vi "verify parameters in range.vi"(8 "error in (no error)":errorcluster, 11 "Simulated_CCD_Camera in":refnum<class "Simulated_CCD_Camera.lvclass">) -> (0 "error out":errorcluster, 3 "Simulated_CCD_Camera out":refnum<class "Simulated_CCD_Camera.lvclass">)   [LabVIEW 2018, in "Simulated_CCD_Camera.lvclass"]
uses:
  Simulated_CCD_Camera.lvclass
  Simulated_CCD_Camera.lvclass/Simulated_CCD_Camera.ctl
  <vilib>/ErrorRing/Error Ring.xnode
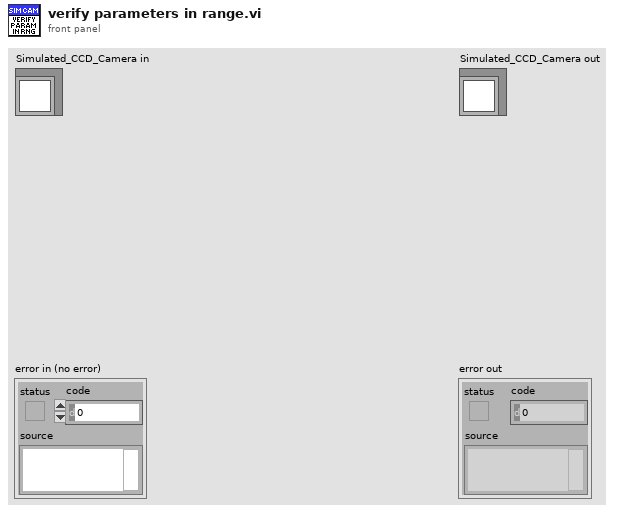
[diagram p1: front panel]
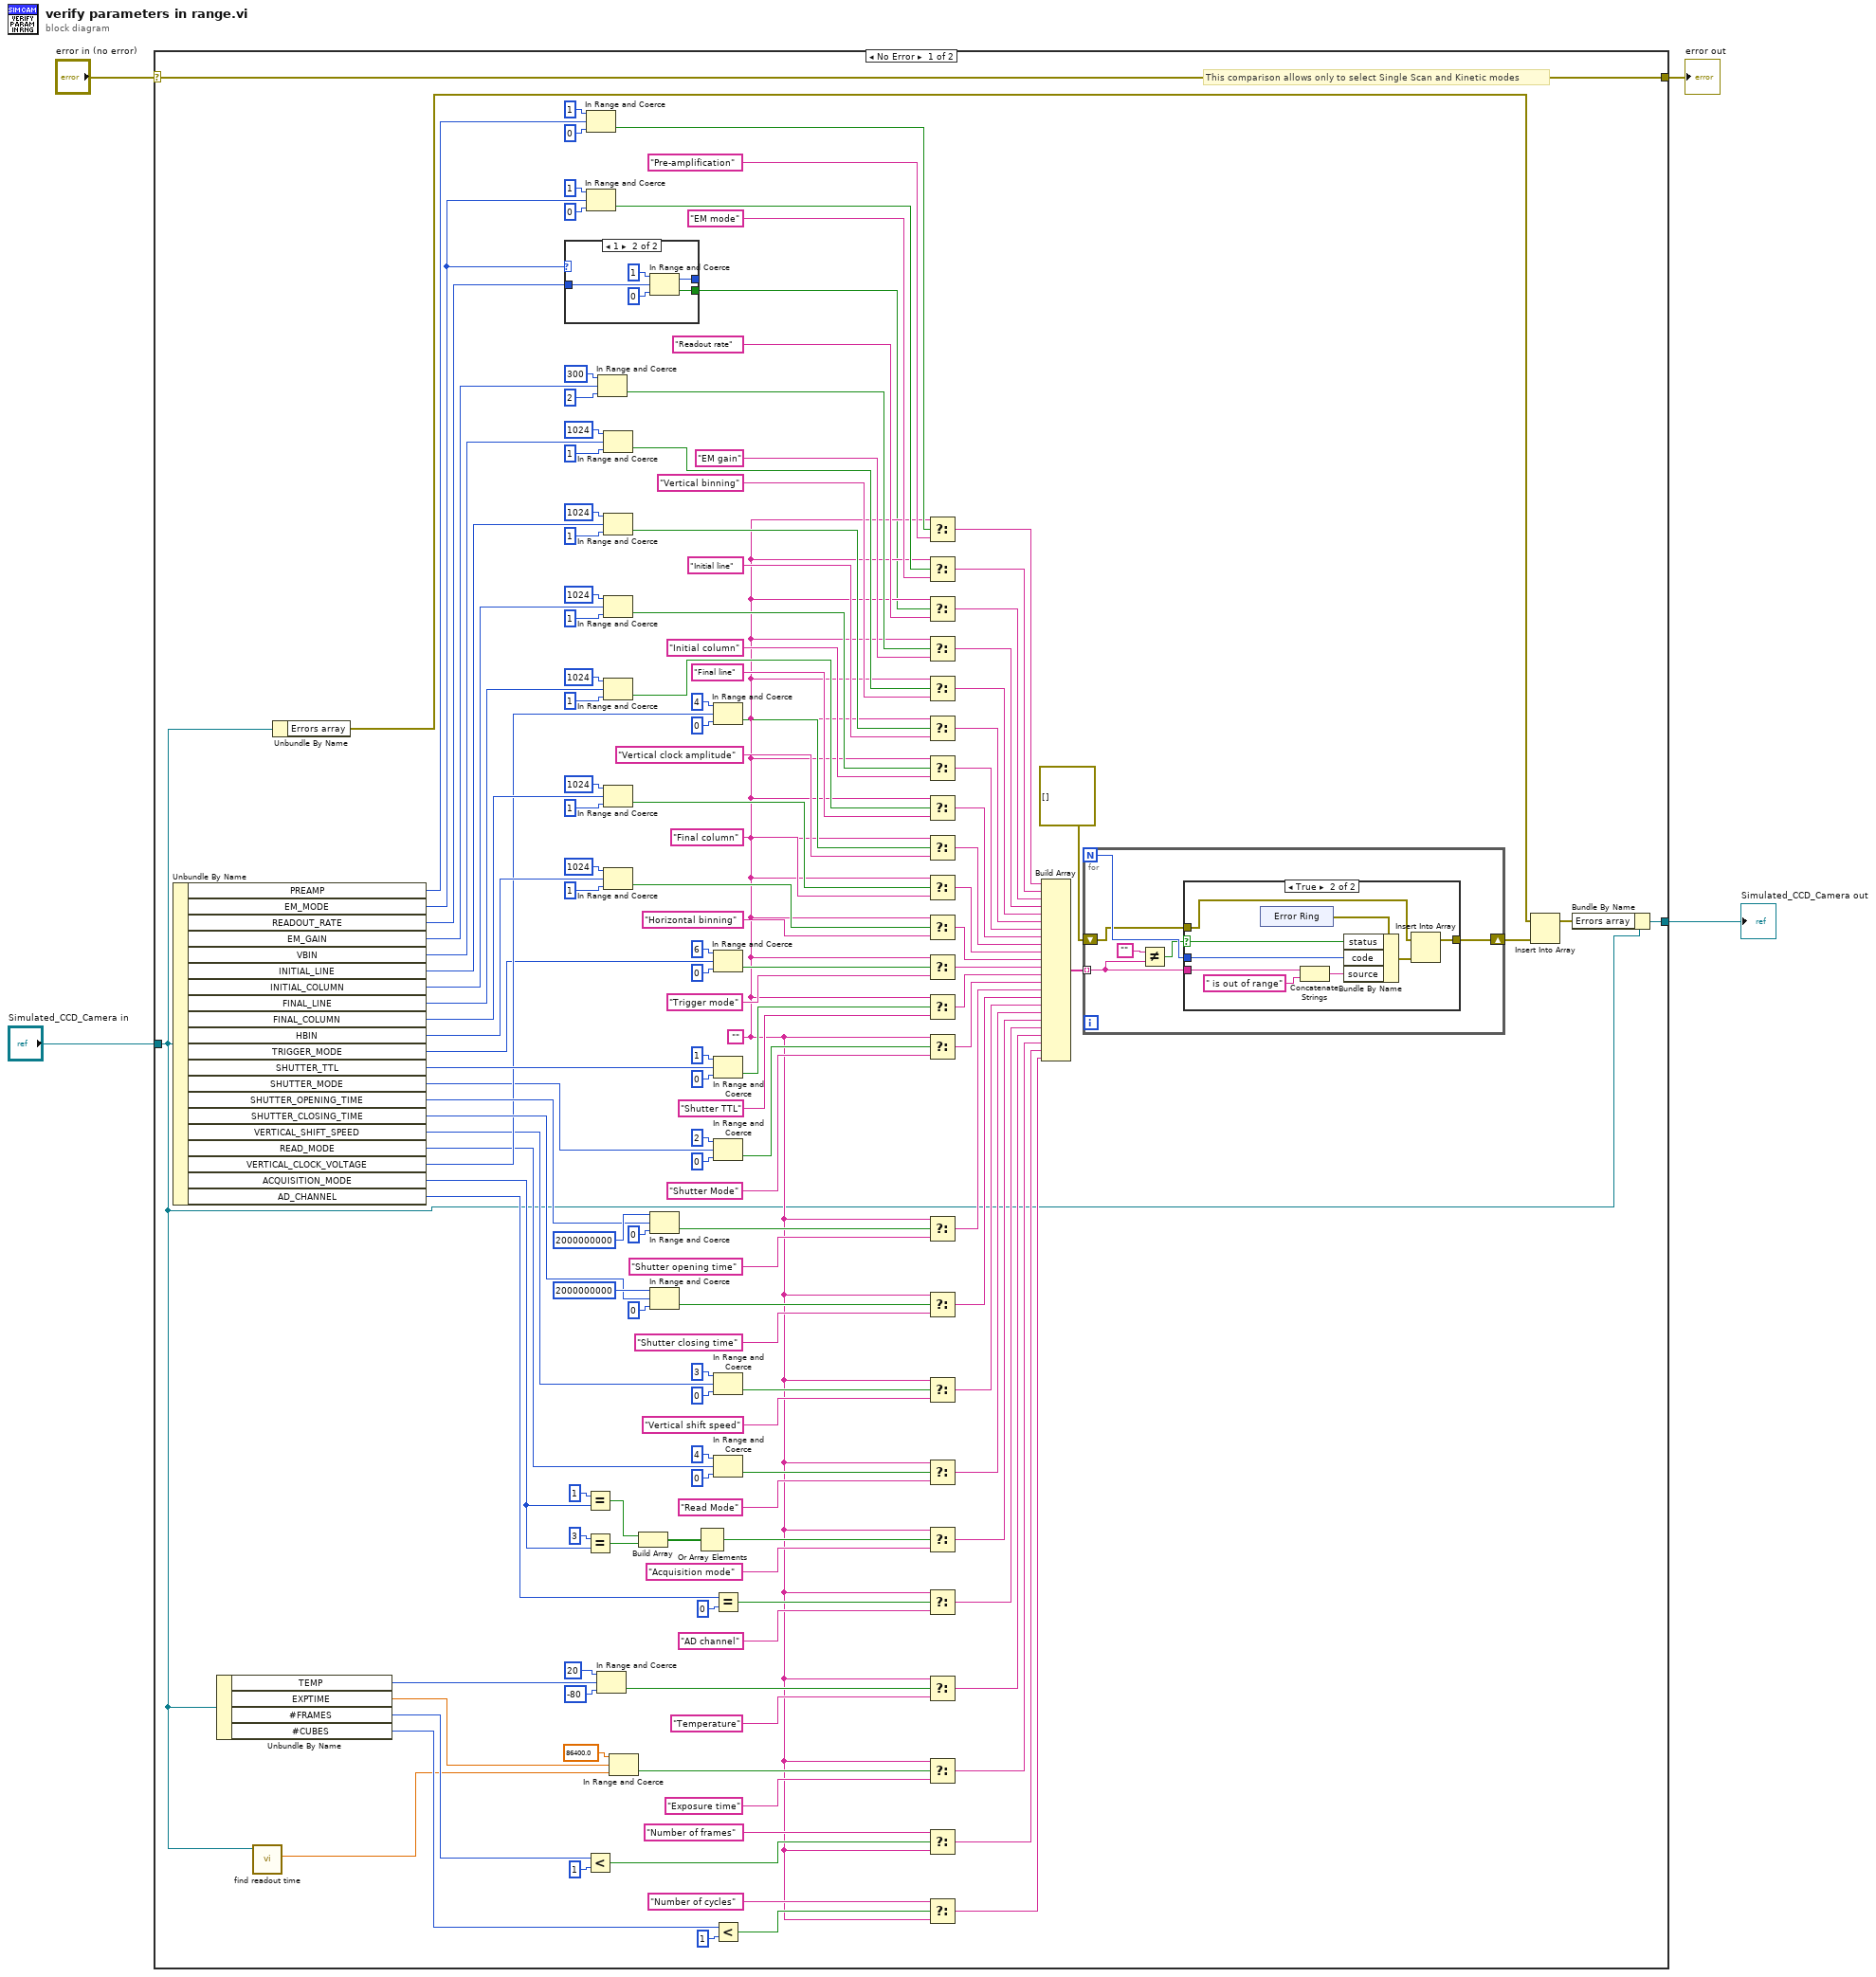
[diagram p0: block diagram]
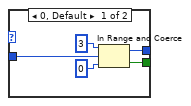
[diagram p3: hidden frame]
diagram:
  n1 = case shown="No Error" "error in (no error)" {
    selector: "error in (no error)" -> [w102 w184]
    tunnel: [w102 w184] -> w3
    tunnel: [w14 w183] -> w1
    tunnel: "Simulated_CCD_Camera in" -> [w6 w183]
    frame No Error {
      w15 = ""
      # "This comparison allows only to select Single Scan and Kinetic modes"
      n2 = Unbundle By Name(w6) -> ("PREAMP"=w153:u16, "EM_MODE"=w150:u16, "READOUT_RATE"=w149:u16, "EM_GAIN"=w146:u16, "VBIN"=w143:u16, "INITIAL_LINE"=w140:u16, "INITIAL_COLUMN"=w137:u16, "FINAL_LINE"=w134:u16, "FINAL_COLUMN"=w131:u16, "HBIN"=w128:u16, "TRIGGER_MODE"=w103:u16, "SHUTTER_TTL"=w125:u16, "SHUTTER_MODE"=w111:u16, "SHUTTER_OPENING_TIME"=w122:u16, "SHUTTER_CLOSING_TIME"=w119:u16, "VERTICAL_SHIFT_SPEED"=w108:u16, "READ_MODE"=w105:u16, "VERTICAL_CLOCK_VOLTAGE"=w116:u16, "ACQUISITION_MODE"=w49:u16, "AD_CHANNEL"=w41:u16)
      n3 = Unbundle By Name(w6) -> ("TEMP"=w34:i32, "EXPTIME"=w29:dbl, "#FRAMES"=w25:u32, "#CUBES"=w20:u32)
      n4 = call "find readout time.vi"("Simulated_CCD_Camera in"=w6) -> ("readout time"=w5:dbl)  [unwired: 8 in, 2 out]
      n5 = Unbundle By Name(w6) -> ("Errors array"=w10:errorcluster[])
      n6 = case shown="1" w150 {
        tunnel: w149 -> [w175 w180]
        tunnel: [w174 w179] -> _
        tunnel: [w173 w178] -> w7
        frame 0, Default {
          n7 = In Range and Coerce(upper limit=3, x=w175, lower limit=0) -> (coerced(x)=w174:i32, In Range?=w173:bool)
        }
        frame 1 {
          n8 = In Range and Coerce(upper limit=1, x=w180, lower limit=0) -> (coerced(x)=w179:i32, In Range?=w178:bool)
        }
      }
      n9 = Equal?(x=1, y=w49) -> (x = y?=w46:bool)
      n10 = Equal?(x=3, y=w49) -> (x = y?=w47:bool)
      n11 = Less?(x=w25, y=1) -> (x < y?=w23:bool)
      n12 = In Range and Coerce(upper limit=1, x=w153, lower limit=0) -> (In Range?=w97:bool)  [unwired: 1 out]
      n13 = In Range and Coerce(upper limit=1, x=w150, lower limit=0) -> (In Range?=w96:bool)  [unwired: 1 out]
      n14 = In Range and Coerce(upper limit=20, x=w34, lower limit=-80) -> (In Range?=w33:bool)  [unwired: 1 out]
      n15 = In Range and Coerce(upper limit=300, x=w146, lower limit=2) -> (In Range?=w93:bool)  [unwired: 1 out]
      n16 = In Range and Coerce(upper limit=1024, x=w143, lower limit=1) -> (In Range?=w90:bool)  [unwired: 1 out]
      n17 = In Range and Coerce(upper limit=1024, x=w140, lower limit=1) -> (In Range?=w85:bool)  [unwired: 1 out]
      n18 = In Range and Coerce(upper limit=1024, x=w137, lower limit=1) -> (In Range?=w84:bool)  [unwired: 1 out]
      n19 = In Range and Coerce(upper limit=1024, x=w134, lower limit=1) -> (In Range?=w81:bool)  [unwired: 1 out]
      n20 = In Range and Coerce(upper limit=1024, x=w131, lower limit=1) -> (In Range?=w77:bool)  [unwired: 1 out]
      n21 = In Range and Coerce(upper limit=1024, x=w128, lower limit=1) -> (In Range?=w74:bool)  [unwired: 1 out]
      n22 = In Range and Coerce(upper limit=86400.0, x=w29, lower limit=w5) -> (In Range?=w28:bool)  [unwired: 1 out]
      n23 = Build Array(w46, w47) -> (w45:bool[])
      n24 = In Range and Coerce(upper limit=2000000000, x=w122, lower limit=0) -> (In Range?=w62:bool)  [unwired: 1 out]
      n25 = In Range and Coerce(upper limit=2000000000, x=w119, lower limit=0) -> (In Range?=w59:bool)  [unwired: 1 out]
      n26 = Or Array Elements(Boolean array=w45) -> (logical OR=w44:bool)
      n27 = In Range and Coerce(upper limit=4, x=w116, lower limit=0) -> (In Range?=w51:bool)  [unwired: 1 out]
      n28 = In Range and Coerce(upper limit=6, x=w103, lower limit=0) -> (In Range?=w72:bool)  [unwired: 1 out]
      n29 = In Range and Coerce(upper limit=1, x=w125, lower limit=0) -> (In Range?=w69:bool)  [unwired: 1 out]
      n30 = In Range and Coerce(upper limit=2, x=w111, lower limit=0) -> (In Range?=w66:bool)  [unwired: 1 out]
      n31 = In Range and Coerce(upper limit=3, x=w108, lower limit=0) -> (In Range?=w57:bool)  [unwired: 1 out]
      n32 = In Range and Coerce(upper limit=4, x=w105, lower limit=0) -> (In Range?=w54:bool)  [unwired: 1 out]
      n33 = Equal?(x=w41, y=0) -> (x = y?=w39:bool)
      n34 = Less?(x=w20, y=1) -> (x < y?=w19:bool)
      n35 = Select(t=w15, s=w97, f="Pre-amplification") -> (s? t:f=w99:string)
      n36 = Select(t=w15, s=w96, f="EM mode") -> (s? t:f=w98:string)
      n37 = Select(t=w15, s=w7, f="Readout rate") -> (s? t:f=w94:string)
      n38 = Select(t=w15, s=w93, f="EM gain") -> (s? t:f=w91:string)
      n39 = Select(t=w15, s=w90, f="Vertical binning") -> (s? t:f=w88:string)
      n40 = Select(t=w15, s=w85, f="Initial line") -> (s? t:f=w86:string)
      n41 = Select(t=w15, s=w84, f="Initial column") -> (s? t:f=w82:string)
      n42 = Select(t=w15, s=w81, f="Final line") -> (s? t:f=w79:string)
      n43 = Select(t=w15, s=w51, f="Vertical clock amplitude") -> (s? t:f=w11:string)
      n44 = Select(t=w15, s=w77, f="Final column") -> (s? t:f=w76:string)
      n45 = Select(t=w15, s=w74, f="Horizontal binning") -> (s? t:f=w73:string)
      n46 = Select(t=w15, s=w72, f="Trigger mode") -> (s? t:f=w70:string)
      n47 = Select(t=w15, s=w69, f="Shutter TTL") -> (s? t:f=w67:string)
      n48 = Select(t=w15, s=w66, f="Shutter Mode") -> (s? t:f=w64:string)
      n49 = Select(t=w15, s=w62, f="Shutter opening time") -> (s? t:f=w61:string)
      n50 = Select(t=w15, s=w59, f="Shutter closing time") -> (s? t:f=w58:string)
      n51 = Select(t=w15, s=w57, f="Vertical shift speed") -> (s? t:f=w55:string)
      n52 = Select(t=w15, s=w54, f="Read Mode") -> (s? t:f=w52:string)
      n53 = Select(t=w15, s=w44, f="Acquisition mode") -> (s? t:f=w42:string)
      n54 = Select(t=w15, s=w39, f="AD channel") -> (s? t:f=w37:string)
      n55 = Select(t=w15, s=w33, f="Temperature") -> (s? t:f=w31:string)
      n56 = Select(t=w15, s=w28, f="Exposure time") -> (s? t:f=w26:string)
      n57 = Select(t="Number of frames" ("f"), s=w23, f=w15) -> (s? t:f=w22:string)
      n58 = Select(t="Number of cycles" ("f"), s=w19, f=w15) -> (s? t:f=w18:string)
      n59 = Build Array(w99, w98, w94, w91, w88, w86, w82, w79, w11, w76, w73, w70, w67, w64, w61, w58, w55, w52, w42, w37, w31, w26, w22, w18) -> (w12:string[])
      n60 = for {
        N -> [w161]
        shift-right: [w160] -> w8
        shift-left: errorcluster[] [] -> [w159]
        tunnel: w12 -> [w156] mode=indexing
        n61 = Not Equal?(x="", y=w156) -> (x != y?=w157:bool)
        n62 = case shown="True" w157 {
          selector: w157 -> [_ w171]
          tunnel: w161 -> [_ w170]
          tunnel: [w162 w169] -> w160
          tunnel: w159 -> [w162 w167]
          tunnel: w156 -> [_ w165]
          frame False {
          }
          frame True {
            n63 = xnode "Error Ring"() -> ("error out"=w168:errorcluster)
            n64 = Concatenate Strings(w165, " is out of range" ("string")) -> (w163:string)
            n65 = Bundle By Name(cluster=w168, "status"=w171, "code"=w170, "source"=w163) -> (w166:errorcluster)
            n66 = Insert Into Array(array=w167, new element=w166) -> (w169:errorcluster[])  [unwired: 1 in]
          }
        }
      }
      n67 = Insert Into Array(array=w10, new element=w8) -> (w9:errorcluster[])  [unwired: 1 in]
      n68 = Bundle By Name(cluster=w6, "Errors array"=w9) -> (w14:refnum<class "Simulated_CCD_Camera.lvclass">)
    }
    frame Error {
    }
  }
  "error out" <- w3
  "Simulated_CCD_Camera out" <- w1
